vi "ReadWrite Channels.vi"(4 "ScheduledSDI":bool, 6 "Iteration":i32, 7 "Mode":T18, 8 "error in (no error)":errorcluster, 9 "SEA9811_RT_data In":T1 {"Tx"."Tx Refs (Data,Trig)"."Data Reference" format="%.0x"}, 10 "FIFOs In":T19, 11 "Channels In":T8[](array[typedef]) {"Labels Settings"."Label" format="%.0o"}) -> (0 "error out":errorcluster, 1 "SEA9811_RT_data Out":T1 {"Tx"."Tx Refs (Data,Trig)"."Data Reference" format="%.0x"}, 2 "FIFOs Out":T19, 3 "Channels Out":T8[](array[typedef]) {"Labels Settings"."Label" format="%.0o"})   [LabVIEW 2012, in "AIT 429 Engine.lvlib"]
uses:
  AIT 429 Engine.lvlib
  RT Controls/FIFO.ctl
  RT Controls/ReadWrite Selector.ctl
  RT Controls/RT HW Channel.ctl
  RT Controls/RT Label Settings.ctl
  Shared/Controls and Global/Label.ctl
  Shared/Controls and Global/transferPeriod.ctl
  RT Controls/Driver Data.ctl
  RT Controls/RT Word Settings.ctl
  <vilib>/NI Veristand/Custom Device API/Block Data Reference.ctl
  <vilib>/NI Veristand/Custom Device API/Data Reference.ctl
  RT Controls/RT Param Setting.ctl
  Shared/Controls and Global/Start Bit.ctl
  Shared/Controls and Global/Number of Bits.ctl
  Shared/Controls and Global/TransferType.ctl
  SEA 9811 FPGA driver/RT/Typdefs/SEA9811_RT_data_cluster.ctl
  <userlib>/_FPGA Interface Advanced Tools/FPGA Interface Base/FPGA Interface Base.lvclass
  SEA 9811 FPGA driver/RT/Typdefs/FPGA ref.ctl
  SEA 9811 FPGA driver/RT/Typdefs/channel.ctl
  SEA 9811 FPGA driver/RT/Typdefs/received word.ctl
  SEA 9811 FPGA driver/RT/Typdefs/SEA9811_FPGA_FP_Addresses.ctl
  Read incoming label data.vi
  Read Parameter VS Channels.vi
  Update Parameter VS Channels.vi
  Shared/Word to double.vi
  <vilib>/NI Veristand/Custom Device API/NI VeriStand - Get Channel Values by Block Data Reference.vi
  <vilib>/NI Veristand/Custom Device API/NI VeriStand - Set Channel Values by Block Data Reference.vi
  <vilib>/NI Veristand/Custom Device API/Global Data Refs.vi
  <instrlib>/AIT 429/AIT 429.lvlib
  <userlib>/ARINC-429/Owl429.lvlib
  Shared/ARINC 429 Shared.lvlib
  <vilib>/NI Veristand/Custom Device API/Custom Device API.lvlib
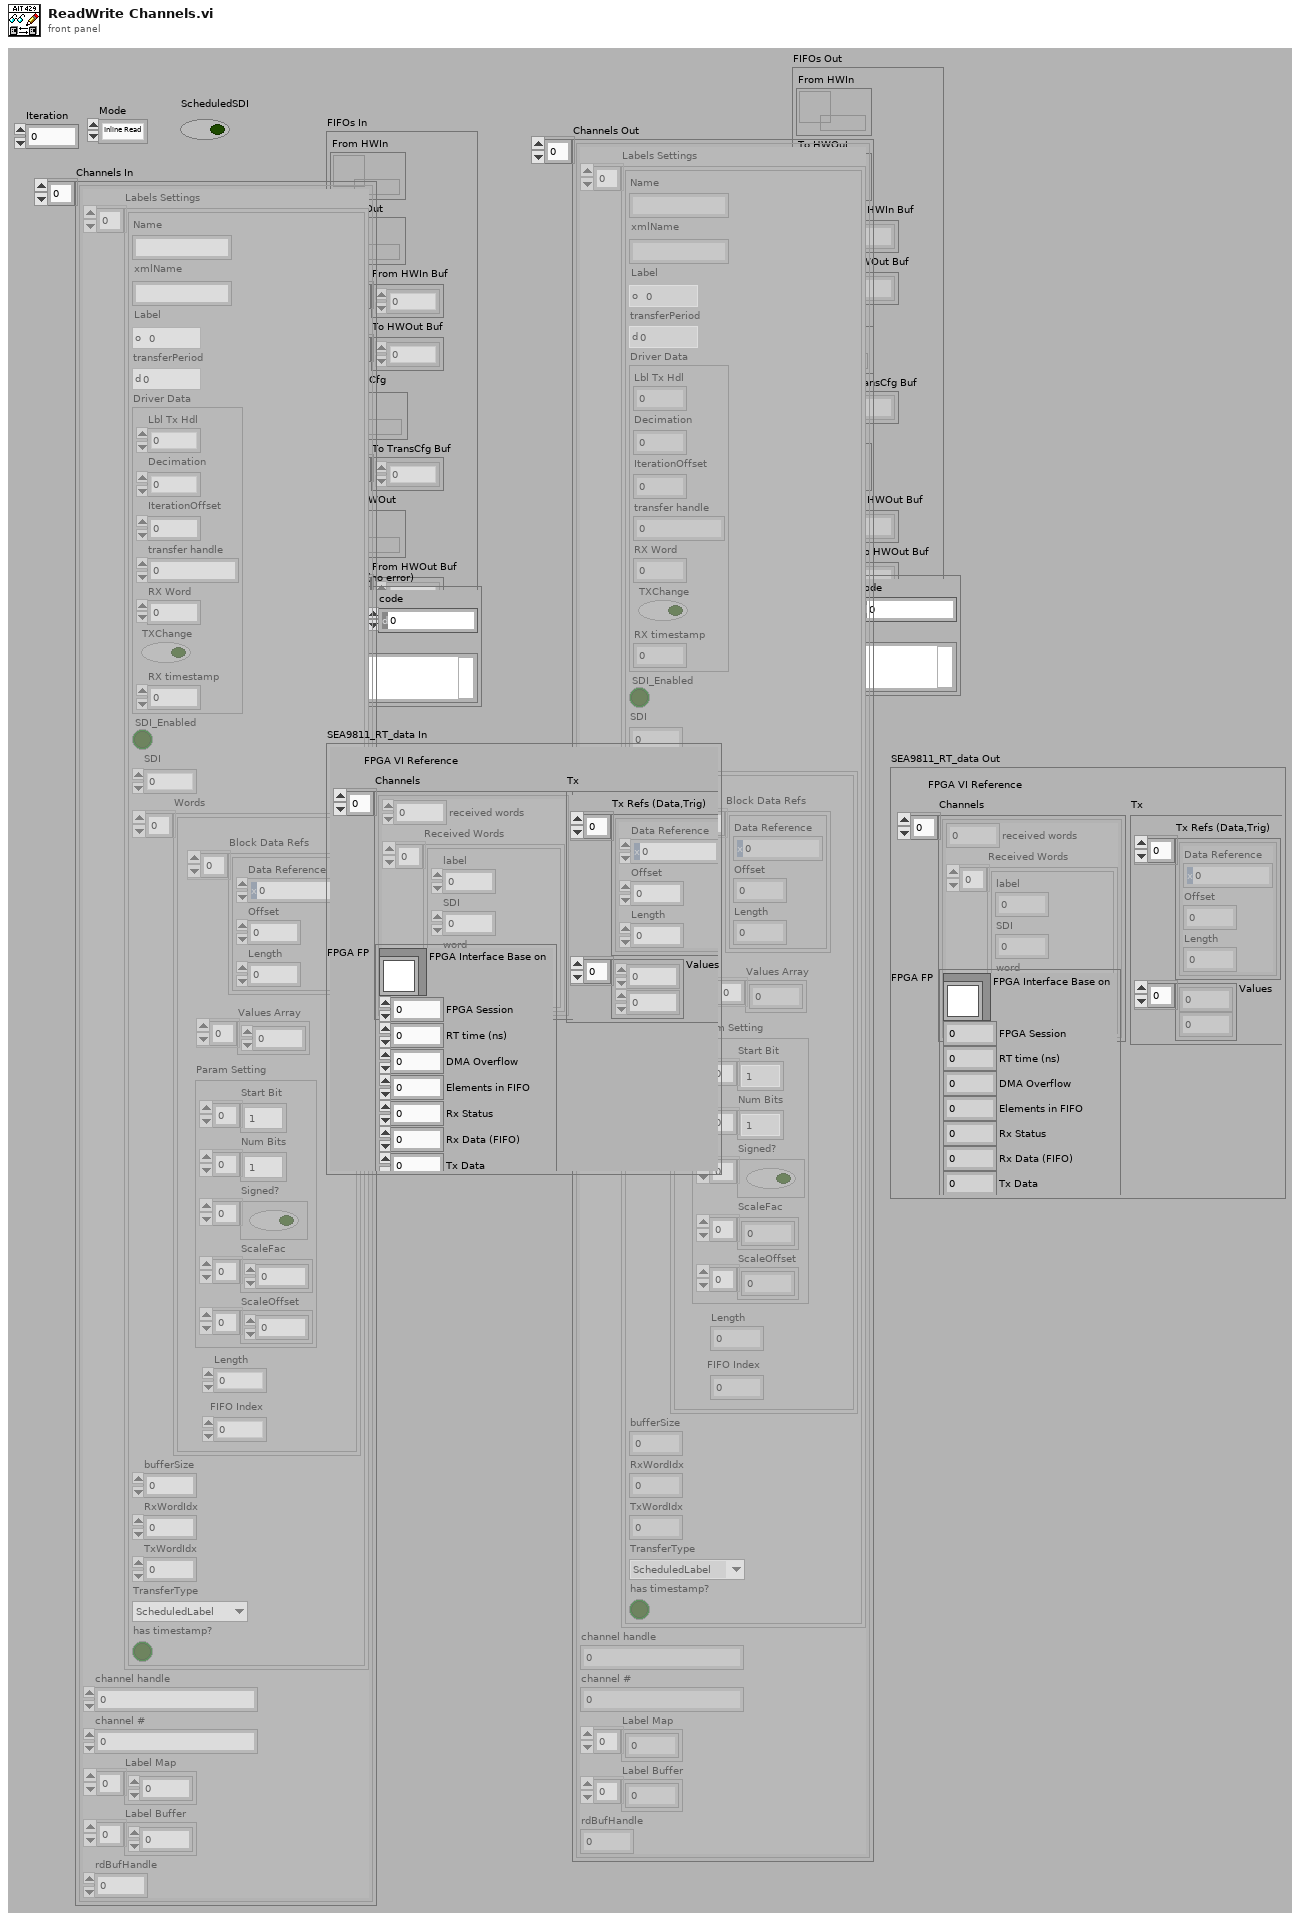
[diagram p1: front panel]
types:
  T1 = typedef "SEA9811_RT_data_cluster.ctl" = cluster{"FPGA VI Reference":T2, "Channels":T3[], "FPGA FP":T5, "Tx":cluster{"Tx Refs (Data,Trig)":T6[], "Values":dbl[]}}
  T2 = typedef "FPGA ref.ctl" = refnum<k20>
  T3 = typedef "channel.ctl" = cluster{"received words":u32, "Received Words":T4[]}
  T4 = typedef "received word.ctl" = cluster{"label":u8, "SDI":u8, "word":u32, "timestamp":dbl}
  T5 = typedef "SEA9811_FPGA_FP_Addresses.ctl" = cluster{"FPGA Interface Base on":refnum<class "FPGA Interface Base.lvclass">, "FPGA Session":u32, "RT time (ns)":u32, "DMA Overflow":u32, "Elements in FIFO":u32, "Rx Status":u32, "Rx Data (FIFO)":u32, "Tx Data":u32, "Transmit Data":u32}
  T6 = typedef "Custom Device API.lvlib/Block Data Reference.ctl" = cluster{"Data Reference":T7, "Offset":i32, "Length":i32}
  T7 = typedef "Custom Device API.lvlib/Data Reference.ctl" = i32
  T8 = typedef "AIT 429 Engine.lvlib/RT HW Channel.ctl" = cluster{"Labels Settings":T9[], "channel handle":u32, "channel #":u16, "Label Map":i32[], "Label Buffer":u32[], "rdBufHandle":u32}
  T9 = typedef "AIT 429 Engine.lvlib/RT Label Settings.ctl" = cluster{"Name":string, "xmlName":string, "Label":T10, "transferPeriod":T11, "Driver Data":T12, "SDI_Enabled":bool, "SDI":u8, "Words":T13[], "bufferSize":u32, "RxWordIdx":i32, "TxWordIdx":i32, "TransferType":T17, "has timestamp?":bool}
  T10 = typedef "ARINC 429 Shared.lvlib/Label.ctl" = u8
  T11 = typedef "ARINC 429 Shared.lvlib/transferPeriod.ctl" = u32
  T12 = typedef "AIT 429 Engine.lvlib/Driver Data.ctl" = cluster{"Lbl Tx Hdl":u32, "Decimation":i32, "IterationOffset":i32, "transfer handle":u32, "RX Word":u32, "TXChange":bool, "RX timestamp":dbl}
  T13 = typedef "AIT 429 Engine.lvlib/RT Word Settings.ctl" = cluster{"Block Data Refs":T6[], "Values Array":dbl[], "Length":i32, "FIFO Index":i32, "Param Setting":T14}
  T14 = typedef "AIT 429 Engine.lvlib/RT Param Setting.ctl" = cluster{"Start Bit":T15[], "Num Bits":T16[], "Signed?":bool[], "ScaleFac":dbl[], "ScaleOffset":dbl[]}
  T15 = typedef "ARINC 429 Shared.lvlib/Start Bit.ctl" = i32
  T16 = typedef "ARINC 429 Shared.lvlib/Number of Bits.ctl" = i32
  T17 = typedef "ARINC 429 Shared.lvlib/TransferType.ctl" = enum16{"ScheduledLabel", "Acyclic", "Block", "Strobe"}
  T18 = typedef "AIT 429 Engine.lvlib/ReadWrite Selector.ctl" = enum16{"Inline Read", "Inline Write", "Async HWIn", "Async HWOut"}
  T19 = typedef "AIT 429 Engine.lvlib/FIFO.ctl" = cluster{"From HWIn":refnum<k33>, "To HWOut":refnum<k33>, "From HWIn Buf":dbl[], "To HWOut Buf":dbl[], "To TansCfg":refnum<k33>, "To TransCfg Buf":dbl[], "From HWOut":refnum<k33>, "From HWOut Buf":dbl[], "Old To HWOut Buf":dbl[]}
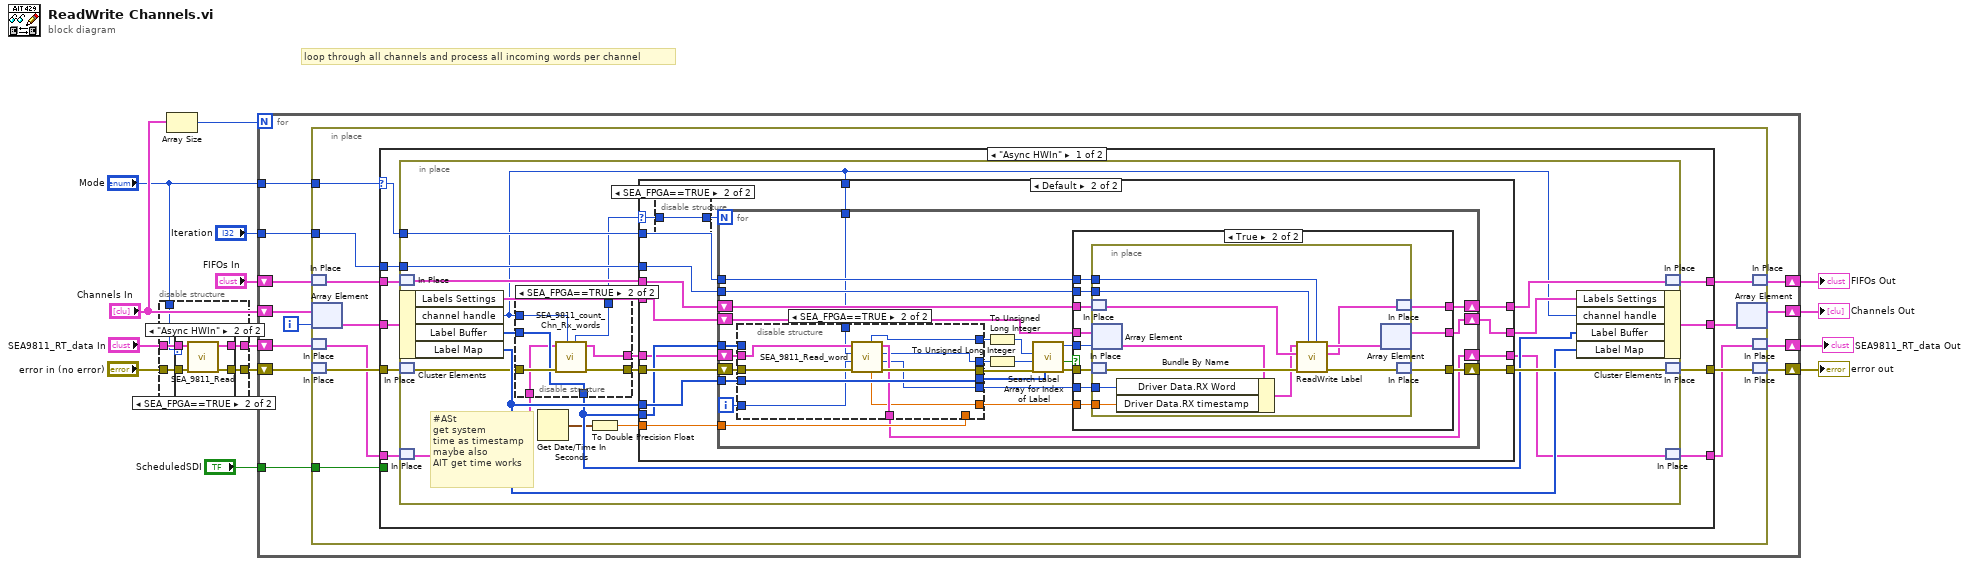
[diagram p0: block diagram]
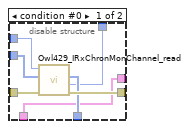
[diagram p4: hidden frame]
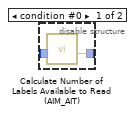
[diagram p6: hidden frame]
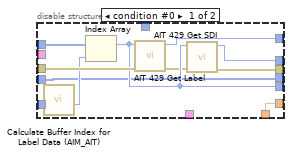
[diagram p7: hidden frame]
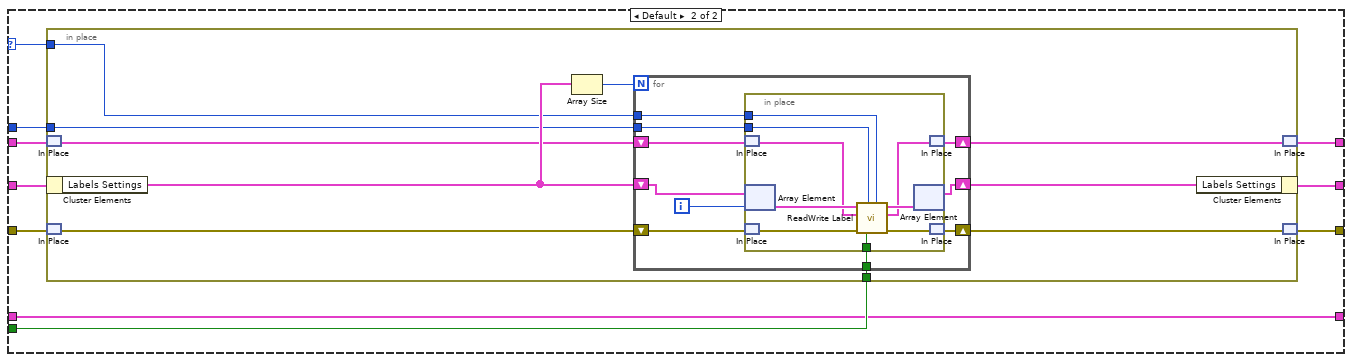
[diagram p9: hidden frame]
diagram:
  # "loop through all channels and process all incoming words per channel"
  n1 = disable-structure shown="SEA_FPGA==TRUE" {
    disable-tunnel: "error in (no error)" -> [w15 w21]
    disable-tunnel: [w15 w20] -> w5
    disable-tunnel: "SEA9811_RT_data In" -> [w16 w19]
    disable-tunnel: [w16 w18] -> w3
    disable-tunnel: "Mode" -> [_ w17]
    frame condition #0 {
    }
    frame condition #1 (active) {
      n2 = case shown="\"Async HWIn\"" w17 {
        tunnel: w21 -> [w22 w27]
        tunnel: [w22 w26] -> w20
        tunnel: w19 -> [w23 w25]
        tunnel: [w23 w24] -> w18
        frame Default {
        }
        frame "Async HWIn" {
          n3 = call "SEA_9811_Read.vi"("error in (no error)"=w27, "SEA9811_RT_data in"=w25) -> ("error out"=w26:errorcluster, "SEA9811_RT_data out"=w24:T1)  [unwired: 6 in, 2 out]
        }
      }
    }
  }
  n4 = Array Size(array="Channels In") -> (size(s)=w9:i32)
  n5 = for {
    N: w9 -> [_]
    shift-right: [w36] -> w12
    shift-left: w5 -> [w37]
    tunnel: "Mode" -> [w35]
    tunnel: "Iteration" -> [w32]
    shift-right: [w38] -> w11
    shift-left: "Channels In" -> [w39]
    shift-right: [w33] -> w14
    shift-left: "FIFOs In" -> [w34]
    tunnel: "ScheduledSDI" -> [w31]
    shift-right: [w29] -> w2
    shift-left: w3 -> [w30]
    i -> [w28]
    n6 = in-place {
      in-place-border: w35 -> [w43]
      in-place-border: w32 -> [w44]
      in-place-border: w31 -> [w42]
      n7 = in-place-match #1(w34) -> (w46:T19)
      n8 = in-place-array #2(w39, w28) -> (w50:T8)
      n9 = in-place-match #3(w30) -> (w41:T1)
      n10 = in-place-match #4(w37) -> (w48:errorcluster)
      n11 = case shown="\"Async HWIn\"" w43 {
        selector: w43 -> [w53 w192]
        tunnel: w50 -> [w60 w199]
        tunnel: [w59 w198] -> w49
        tunnel: w48 -> [w58 w197]
        tunnel: [w57 w196] -> w47
        tunnel: w46 -> [w56 w195]
        tunnel: [w55 w194] -> w45
        tunnel: w44 -> [w54 w193]
        tunnel: w42 -> [_ w191]
        tunnel: w41 -> [w52 w190]
        tunnel: [w51 w190] -> w40
        frame "Async HWIn" {
          n12 = in-place {
            in-place-border: w53 -> [w77]
            in-place-border: w54 -> [w75]
            # "#ASt\nget system\ntime as timestamp\nmaybe also\nAIT get time works"
            n13 = in-place-match #5(w56) -> (w74:T19)
            n14 = in-place-cluster #6(w60) -> ("Labels Settings"=w67:T9[], "channel handle"=w61:u32, "Label Buffer"=w68:u32[], "Label Map"=w73:i32[])
            n15 = in-place-match #7(w58) -> (w71:errorcluster)
            n16 = in-place-match #8(w52) -> (w64:T1)
            n17 = disable-structure shown="SEA_FPGA==TRUE" {
              disable-tunnel: [w86 w92] -> w72
              disable-tunnel: w71 -> [w85 w93]
              disable-tunnel: w61 -> [w84 w90]
              disable-tunnel: [w83 w89] -> w70
              disable-tunnel: [w82 w91] -> w69
              disable-tunnel: w68 -> [w81 w89]
              disable-tunnel: w64 -> [w80 w88]
              disable-tunnel: [w80 w87] -> w63
              frame condition #0 {
                n18 = call <userlib>:"Owl429_IRxChronMonChannel_read.vi"("error in (no error)"=w85, "data buffer"=w81, "channel handle"=w84) -> ("error out"=w86:errorcluster, "word count"=w82:u32, "data buffer"=w83:u32[])  [unwired: 5 in, 1 out]
              }
              frame condition #1 (active) {
                n19 = call "SEA_9811_count_Chn_Rx_words.vi"("channel #"=w90, "error in (no error)"=w93, "SEA9811_RT_data in"=w88) -> ("error out"=w92:errorcluster, "SEA9811_RT_data out"=w87:T1, "received words"=w91:u32)  [unwired: 6 in]
              }
            }
            n20 = Get Date/Time In Seconds() -> (seconds since 1Jan1904=w66:timestamp)
            n21 = To Double Precision Float(number=w66) -> (double precision float=w65:dbl)
            n22 = case shown="Default" w69 {
              selector: w69 -> [_ w102]
              tunnel: w67 -> [w96 w113]
              tunnel: [w96 w112] -> w79
              tunnel: [w97 w111] -> w78
              tunnel: w77 -> [_ w110]
              tunnel: [w95 w109] -> w76
              tunnel: w75 -> [_ w108]
              tunnel: w74 -> [w95 w107]
              tunnel: w73 -> [_ w106]
              tunnel: w72 -> [w97 w105]
              tunnel: w70 -> [_ w104]
              tunnel: w65 -> [_ w101]
              tunnel: w63 -> [w94 w100]
              tunnel: [w94 w99] -> w62
              tunnel: w61 -> [_ w98]
              frame 0 {
              }
              frame Default {
                n23 = disable-structure shown="SEA_FPGA==TRUE" {
                  disable-tunnel: [w115 w116] -> w103
                  disable-tunnel: w102 -> [w114 w116]
                  frame condition #0 {
                    n24 = call "Calculate Number of Labels Available to Read (AIM_AIT).vi"("entry count"=w114) -> ("# of labels available"=w115:dbl)  [unwired: 10 in]
                  }
                  frame condition #1 (active) {
                  }
                }
                n25 = for {
                  N: w103 -> [_]
                  shift-right: [w141] -> w111
                  shift-left: w105 -> [w136]
                  tunnel: w110 -> [w140]
                  tunnel: w108 -> [w137]
                  tunnel: w104 -> [w132]
                  shift-right: [w138] -> w109
                  shift-left: w107 -> [w139]
                  shift-right: [w142] -> w112
                  shift-left: w113 -> [w135]
                  tunnel: w106 -> [w120]
                  tunnel: w101 -> [w122]
                  shift-right: [w118] -> w99
                  shift-left: w100 -> [w123]
                  tunnel: w98 -> [w117]
                  i -> [w130]
                  n26 = disable-structure shown="SEA_FPGA==TRUE" {
                    disable-tunnel: w136 -> [w153 w162]
                    disable-tunnel: w132 -> [w152 _]
                    disable-tunnel: w130 -> [w151 w155]
                    disable-tunnel: [w149 w158] -> w129
                    disable-tunnel: [w148 w161] -> w128
                    disable-tunnel: [w147 w160] -> w127
                    disable-tunnel: [w146 w157] -> w126
                    disable-tunnel: w123 -> [_ w163]
                    disable-tunnel: w122 -> [w144 _]
                    disable-tunnel: [w144 w156] -> w121
                    disable-tunnel: w120 -> [w143 w164]
                    disable-tunnel: [w143 w164] -> w119
                    disable-tunnel: [_ w159] -> w118
                    disable-tunnel: w117 -> [_ w154]
                    frame condition #0 {
                      n27 = call "Calculate Buffer Index for Label Data (AIM_AIT).vi"("Iteration"=w151) -> ("Buffer index"=w150:u32)  [unwired: 10 in]
                      n28 = Index Array(array=w152, index=w150) -> (element=w146:u32)
                      n29 = call <instrlib>:"AIT 429 Get Label.vi"("error in (no error)"=w153, "word"=w146) -> ("error out"=w145:errorcluster, "label"=w147:u8)  [unwired: 8 in]
                      n30 = call <instrlib>:"AIT 429 Get SDI.vi"("error in (no error)"=w145, "word"=w146) -> ("error out"=w148:errorcluster, "sdi"=w149:u8)  [unwired: 8 in]
                    }
                    frame condition #1 (active) {
                      n31 = call "SEA_9811_Read_word.vi"("error in (no error)"=w162, "i"=w155, "channel #"=w154, "SEA9811_RT_data in"=w163) -> ("error out"=w161:errorcluster, "word"=w157:u32, "SDI"=w158:u8, "SEA9811_RT_data out"=w159:T1, "timestamp"=w156:dbl, "label"=w160:u8)  [unwired: 2 in]
                    }
                  }
                  n32 = To Unsigned Long Integer(number=w127) -> (unsigned 32bit integer=w125:u32)
                  n33 = To Unsigned Long Integer(number=w129) -> (unsigned 32bit integer=w124:u32)
                  n34 = call "Search Label Array for Index of Label.vi"("Label Map"=w119, "error in (no error)"=w128, "sdi"=w124, "label"=w125) -> ("error out"=w133:errorcluster, "Label Found?"=w131:bool, "Index"=w134:i32)  [unwired: 5 in]
                  n35 = case shown="True" w131 {
                    tunnel: [w166 w178] -> w142
                    tunnel: [w165 w177] -> w141
                    tunnel: w140 -> [_ w176]
                    tunnel: w139 -> [w167 w175]
                    tunnel: [w167 w174] -> w138
                    tunnel: w137 -> [_ w173]
                    tunnel: w135 -> [w166 w172]
                    tunnel: w134 -> [_ w171]
                    tunnel: w133 -> [w165 w170]
                    tunnel: w126 -> [_ w169]
                    tunnel: w121 -> [_ w168]
                    frame False {
                    }
                    frame True {
                      n36 = in-place {
                        in-place-border: w176 -> [w186]
                        in-place-border: w173 -> [w185]
                        in-place-border: w169 -> [w180]
                        in-place-border: w168 -> [w179]
                        n37 = in-place-match #9(w175) -> (w184:T19)
                        n38 = in-place-array #10(w172, w171) -> (w182:T9)
                        n39 = in-place-match #11(w170) -> (w189:errorcluster)
                        n40 = Bundle By Name(cluster=w182, "Driver Data.RX Word"=w180, "Driver Data.RX timestamp"=w179) -> (w181:T9)
                        n41 = call "ReadWrite Label.vi"("Mode"=w186, "Iteration"=w185, "error in (no error)"=w189, "FIFOs In"=w184, "Label In"=w181) -> ("error out"=w188:errorcluster, "FIFOs Out"=w183:T19, "Label Out"=w187:T9)  [unwired: 4 in]
                        n42 = in-place-array #10(w187) -> (w178:T9[])  [unwired: 1 out]
                        n43 = in-place-match #9(w183) -> (w174:T19)
                        n44 = in-place-match #11(w188) -> (w177:errorcluster)
                      }
                    }
                  }
                }
              }
            }
            n45 = in-place-cluster #6("Labels Settings"=w79, "channel handle"=w61, "Label Buffer"=w70, "Label Map"=w73) -> (w59:T8)
            n46 = in-place-match #5(w76) -> (w55:T19)
            n47 = in-place-match #7(w78) -> (w57:errorcluster)
            n48 = in-place-match #8(w62) -> (w51:T1)
          }
        }
        frame Default {
          n49 = in-place {
            in-place-border: w192 -> [w205]
            in-place-border: w193 -> [w203]
            in-place-border: w191 -> [w200]
            n50 = in-place-match #12(w195) -> (w202:T19)
            n51 = in-place-cluster #13(w199) -> ("Labels Settings"=w208:T9[])
            n52 = in-place-match #14(w197) -> (w201:errorcluster)
            n53 = Array Size(array=w208) -> (size(s)=w209:i32)
            n54 = for {
              N: w209 -> [_]
              shift-right: [w215] -> w206
              shift-left: w201 -> [w216]
              tunnel: w205 -> [w214]
              tunnel: w203 -> [w211]
              shift-right: [w212] -> w204
              shift-left: w202 -> [w213]
              shift-right: [w217] -> w207
              shift-left: w208 -> [w219]
              tunnel: w200 -> [w210]
              i -> [w218]
              n55 = in-place {
                in-place-border: w214 -> [w225]
                in-place-border: w211 -> [w226]
                in-place-border: w210 -> [w220]
                n56 = in-place-match #15(w213) -> (w221:T19)
                n57 = in-place-array #16(w219, w218) -> (w222:T9)
                n58 = in-place-match #17(w216) -> (w223:errorcluster)
                n59 = call "ReadWrite Label.vi"("Mode"=w225, "ScheduledSDI"=w220, "Iteration"=w226, "error in (no error)"=w223, "FIFOs In"=w221, "Label In"=w222) -> ("error out"=w228:errorcluster, "FIFOs Out"=w224:T19, "Label Out"=w227:T9)  [unwired: 3 in]
                n60 = in-place-array #16(w227) -> (w217:T9[])  [unwired: 1 out]
                n61 = in-place-match #15(w224) -> (w212:T19)
                n62 = in-place-match #17(w228) -> (w215:errorcluster)
              }
            }
            n63 = in-place-cluster #13("Labels Settings"=w207) -> (w198:T8)
            n64 = in-place-match #12(w204) -> (w194:T19)
            n65 = in-place-match #14(w206) -> (w196:errorcluster)
          }
        }
      }
      n66 = in-place-array #2(w49) -> (w38:T8[])  [unwired: 1 out]
      n67 = in-place-match #1(w45) -> (w33:T19)
      n68 = in-place-match #3(w40) -> (w29:T1)
      n69 = in-place-match #4(w47) -> (w36:errorcluster)
    }
  }
  "FIFOs Out" <- w14
  "error out" <- w12
  "Channels Out" <- w11
  "SEA9811_RT_data Out" <- w2
